vi "NS Main.vi"(8 "error in (no error)":errorcluster, 11 "Ip Address":string) -> (0 "error out":errorcluster, 3 "Connected  ?":bool)   [LabVIEW 2020]
uses:
  Globals/Phase III Globals.vi
  Controls/NS Data type.ctl
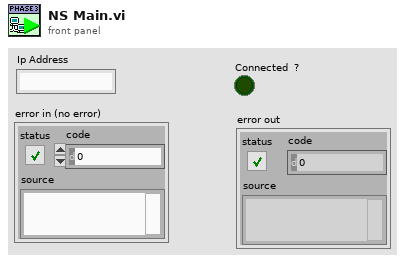
[diagram p1: front panel]
types:
  T1 = typedef "NS Data type.ctl" = cluster{string, variant}
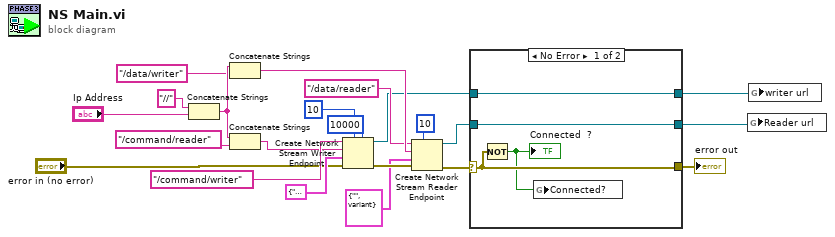
[diagram p0: block diagram]
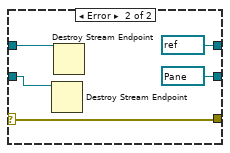
[diagram p2: hidden frame]
diagram:
  n1 = Concatenate Strings("//" ("reader url"), "Ip Address") -> (w20:string)
  n2 = Concatenate Strings(w20, "/data/writer" ("reader url")) -> (w15:string)
  n3 = Concatenate Strings(w20, "/command/reader" ("reader url")) -> (w16:string)
  n4 = Create Network Stream Writer Endpoint(5:10000 ("timeout in ms (-1)"), 7:10 ("timeout in ms (-1)"), 8:"error in (no error)", 9:cluster{string, variant} {"", variant}, 10:w16, 11:"/command/writer" ("writer name")) -> (0:w13:errorcluster, 3:w6:refnum<k21>)  [unwired: 1 in]
  n5 = Create Network Stream Reader Endpoint(7:10 ("reader buffer size"), 8:w13, 9:T1 {"", variant}, 10:w15, 11:"/data/reader" ("writer name")) -> (0:w7:errorcluster, 3:w5:refnum<k21>)  [unwired: 2 in]
  n6 = case shown="No Error" w7 {
    selector: w7 -> [w24 w28]
    tunnel: [w26 refnum<k21> refnum ("writer name")] -> w4
    tunnel: w6 -> [w26 w31]
    tunnel: [w25 refnum<k21> refnum ("writer name")] -> w3
    tunnel: w5 -> [w25 w30]
    tunnel: [w24 w28] -> w2
    frame No Error {
      n7 = Not(x=w24) -> (.not. x?=w23:bool)
      "Connected  ?" <- w23
      n8 = global write "Phase III Globals.vi" "Connected?"(w23) -> ()
    }
    frame Error {
      n9 = Destroy Stream Endpoint(11:w30) -> ()  [unwired: 1 in, 1 out]
      n10 = Destroy Stream Endpoint(11:w31) -> ()  [unwired: 1 in, 1 out]
    }
  }
  "error out" <- w2
  n11 = global write "Phase III Globals.vi" "Reader url"(w3) -> ()
  n12 = global write "Phase III Globals.vi" "writer url"(w4) -> ()
